vi "Online Peak Detection and Display in Strip Mode.vi"() -> ()   [LabVIEW 2023]
doc: "This example shows how to use WA Online Multiscale Peak Detection VI to detect peaks and valleys in a streaming signal and display the result in a graph using strip mode.\n\n<b>Instructions:</b>\n1) Select the <b>Data</b> and <b> Block size</b>. This example will split the input signal into blocks and stream the signal to Online Multiscale Peak Detection VI block-by-block.\n2) Set the <b>Width</b> and other settings for peak detection.\n3) Set the <b>Display block size</b>, which specifies the buffer size for displaying the detection result in strip mode.\n4) Run this VI.\n5) Obseve the peak detection results on the <b>Block View</b>."
uses:
  <vilib>/addons/Wavelet Analysis/online wavelet analysis.llb/WA Online Multiscale Peak Detection (Waveform).vi
  <vilib>/addons/_Advanced Signal Processing/NI_AdvSigProcOnlineWA.lvlib
  <vilib>/addons/_Advanced Signal Processing/NI_AdvSigProcWA.lvlib
panel:
  out "Peak/valley amplitude":dbl[](array[numeric])
  in  "Display block size":i32=900
  out "Block View":cluster{"Ramp Pattern":dbl[], "trend":dbl[]}[](graph)
  out "Peak/valley location":dbl[](array[numeric])
  in  "Peaks/valleys":u16(ring) items=["peaks", "valleys"]
  in  "Block size":i32=180
  in  "Data":u16(ring)=131 items=["1D Example Data"=100, "-"=101, "Doppler"=102, "HOP"=103, "TF Sine"=104, "Noisy Doppler"=105, "Sea Temperature"=106, "Sp500"=107, "Power Line"=108, "Engine Knocking"=109, "HeaviSine"=110, "Bumps"=111, "Blocks"=112, "Piece Regular"=113, "HypChirps"=114, "LinChirps"=115, "Chirps"=116, "Piece Polynomial"=117, "ECG"=131, "-"=118, "2D Example Data"=119, "-"=120, "Finger Print (Image)"=121, "Iris Flower (Image)"=122, "Mammogram (Image)"=123, "Lake (Image)"=127, "Two Can 1 (Image)"=132, "Two Can 2 (Image)"=133, "Camera Man (Image)"=134]
  in  "Detrend settings":T1={"detrend? (F)"=FALSE, "threshold frequency"=-1.0}
  in  "Width":i32=8
  in  "Threshold":dbl=0.5
  # "Overview: Shows how to use WA Online Multiscale Peak Detection VI to detect peaks and valleys in a streaming signal and display the result in a graph using strip mode.\nRequirements: LabVIEW Full Development System, Advanced Signal Processing Toolkit\nInstructions: \n1. Select the Data and  Block size. This example will split the input signal into blocks and stream the signal to Online Multiscale Peak Detection VI block-by-block.\n2. Set the Width and other settings for peak detection.\n3. Set the Display block size, which specifies the buffer size for displaying the detection result in strip mode.\n4. Run this VI.\n5. Observe the peak detection results on the Block View."
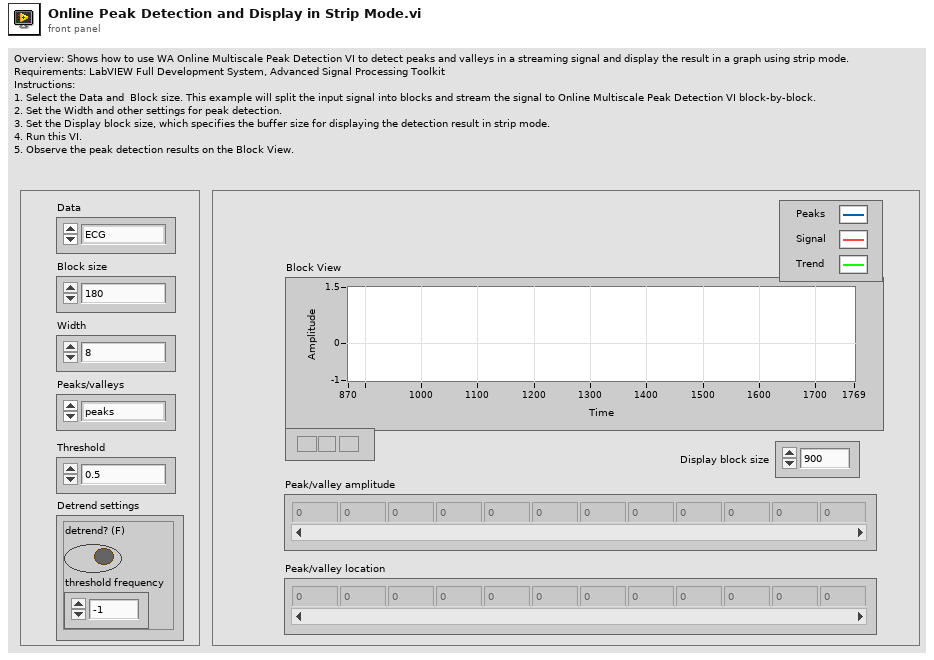
[diagram p1: front panel]
types:
  T1 = cluster{"detrend? (F)":bool, "threshold frequency":dbl}
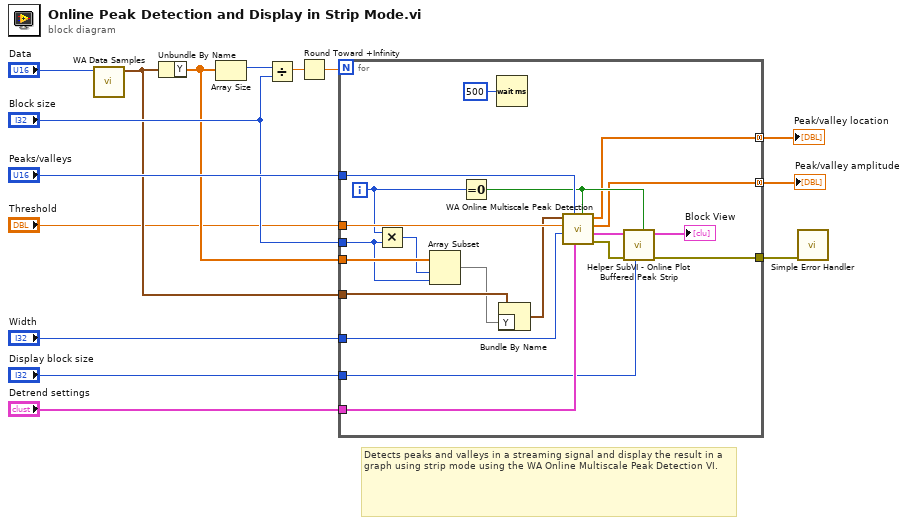
[diagram p0: block diagram]
diagram:
  # "Detects peaks and valleys in a streaming signal and display the result in a graph using strip mode using the WA Online Multiscale Peak Detection VI."
  n1 = call <vilib>:"WA Data Samples.vi"("data"="Data") -> ("signal"=w7:waveform(dbl))  [unwired: 9 in, 1 out]
  n2 = Unbundle By Name(w7) -> ("Y"=w6:dbl[])
  n3 = Array Size(array=w6) -> (size(s)=w13:i32)
  n4 = Divide(x=w13, y="Block size") -> (x/y=w12:dbl)
  n5 = Round Toward +Infinity(x=w12) -> (ceil(x): smallest int >= x=w11:dbl)
  n6 = for {
    N: w11 -> [_]
    tunnel: "Threshold" -> [w35]
    tunnel: "Width" -> [w34]
    tunnel: "Detrend settings" -> [w33]
    tunnel: "Peaks/valleys" -> [w32]
    tunnel: "Display block size" -> [w27]
    tunnel: w6 -> [w26]
    tunnel: "Block size" -> [w23]
    tunnel: w7 -> [w22]
    tunnel: [w18] -> w3
    tunnel: [w17] -> w2 mode=concatenating
    tunnel: [w16] -> w1 mode=concatenating
    i -> [w25]
    n7 = Multiply(x=w25, y=w23) -> (x*y=w24:i32)
    n8 = Array Subset(array=w26, index=w24, length=w23) -> (w21:dbl[])
    n9 = Equal To 0?(x=w25) -> (x = 0?=w28:bool)
    n10 = Wait (ms)(milliseconds to wait=u32 500 ("millisecond multiple")) -> ()  [unwired: 1 out]
    n11 = Bundle By Name(cluster=w22, "Y"=w21) -> (w20:waveform(dbl))
    n12 = call-poly <vilib>:"WA Online Multiscale Peak Detection.vi"("initialize? (F)"=w28, "detrend settings"=w33, "peaks/valleys"=w32, "width"=w34, "threshold"=w35, "signal"=w20) -> ("error out"=w31:errorcluster, "peak plot"=w30:cluster{"Ramp Pattern":dbl[], "X":dbl[]}[], "amplitude"=w16:dbl[], "location"=w17:dbl[])  [unwired: 2 in]
    n13 = call "Helper SubVI - Online Plot Buffered Peak Strip.vi"("initialize? (F)"=w28, "block size"=w27, "error in (no error)"=w31, "peak plot"=w30) -> ("error out"=w18:errorcluster, "plot data"=→"Block View":cluster{"Ramp Pattern":dbl[], "trend":dbl[]}[])  [unwired: 6 in]
  }
  "Peak/valley location" <- w2
  "Peak/valley amplitude" <- w1
  n14 = call <vilib>:"Simple Error Handler.vi"("error in (no error)"=w3) -> ()  [unwired: 4 in, 5 out]
